vi "manipulate files.vi"(8 "error in":errorcluster) -> (0 "error out":errorcluster)   [LabVIEW 2023]
uses:
  queue/Front Panel Message Queue.lvlib
panel:
  in  "Path to Rename":path
  in  "starting number":i32
  in  "Number to bin":i32
  in  "Path to Bin":path
  in  "binning":bool
  in  "rename":bool
  in  "Stop":bool
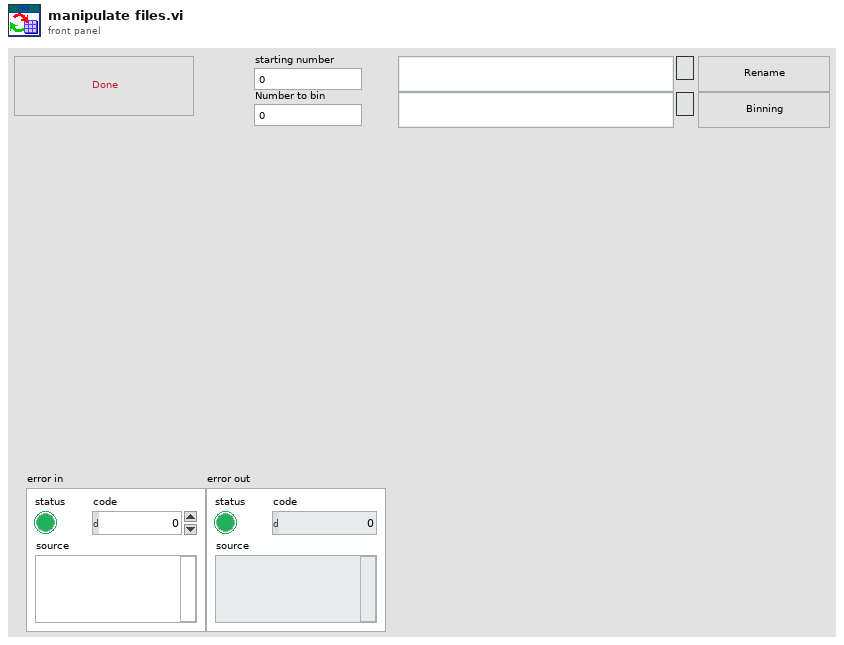
[diagram p1: front panel]
types:
  T1 = typedef "Front Panel Message Queue.lvlib/load Message Queues.ctl" = cluster{"Main":refnum<queue>}
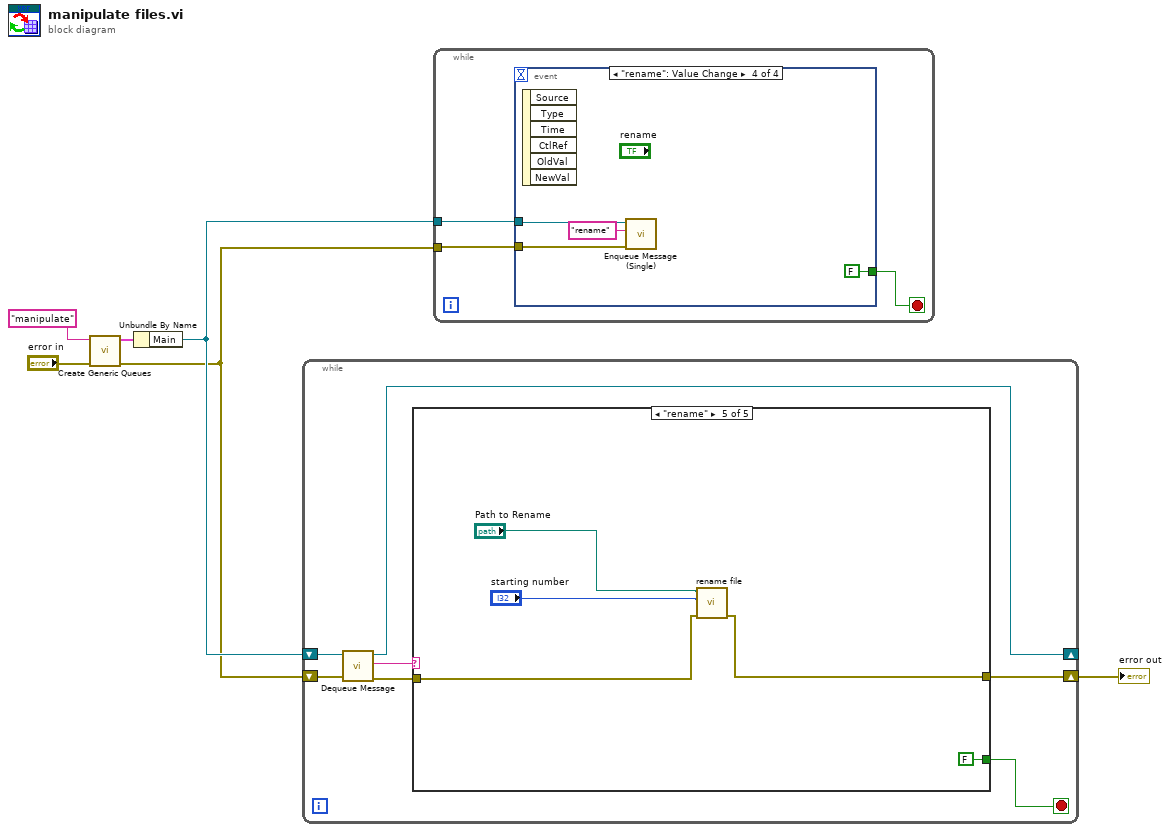
[diagram p0: block diagram]
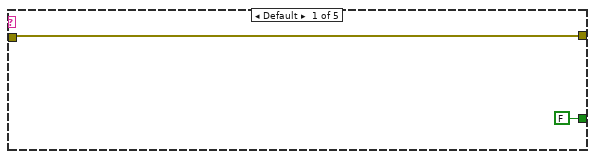
[diagram p2: hidden frame]
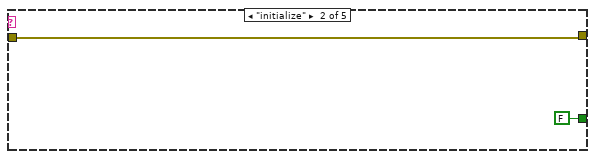
[diagram p3: hidden frame]
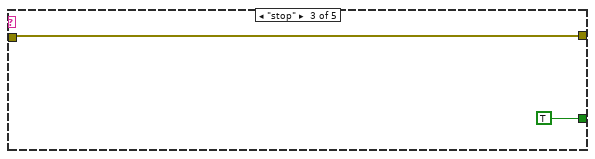
[diagram p4: hidden frame]
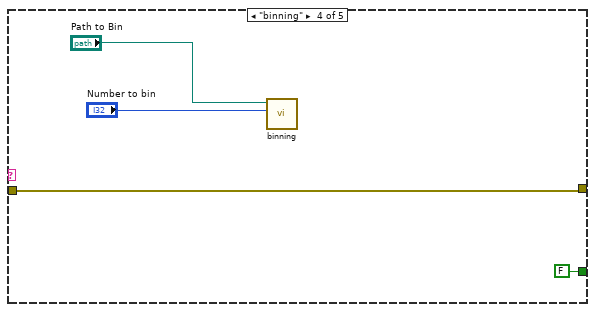
[diagram p5: hidden frame]
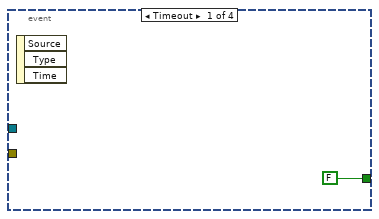
[diagram p6: hidden frame]
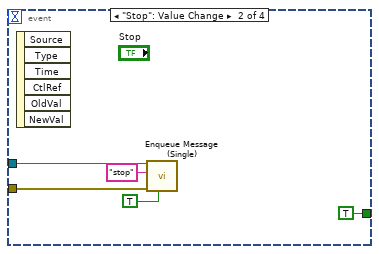
[diagram p7: hidden frame]
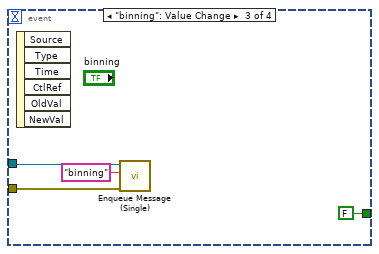
[diagram p8: hidden frame]
diagram:
  n1 = call "Create Generic Queues.vi"("error in (no error)"="error in", "name"="manipulate") -> ("error out"=w2:errorcluster, "Message Queues"=w4:T1)  [unwired: 8 in]
  n2 = Unbundle By Name(w4) -> ("Main"=w3:refnum<queue>)
  n3 = while {
    shift-right: [w10] -> _
    shift-left: w3 -> [w13]
    shift-right: [w9] -> w1
    shift-left: w2 -> [w12]
    stop <- w7 stop-if-true
    n4 = call "Dequeue Message.vi"("error in (no error)"=w12, "Message Queue"=w13) -> ("error out"=w11:errorcluster, "Message"=w8:string, "dup Message Queue"=w10:refnum<queue>)  [unwired: 5 in, 2 out]
    n5 = case shown="\"rename\"" w8 {
      tunnel: w11 -> [w15 w17 w18 w20 w25]
      tunnel: [w15 w17 w18 w20 w24] -> w9
      tunnel: [FALSE FALSE TRUE FALSE FALSE] -> w7
      frame Default {
      }
      frame "initialize" {
      }
      frame "stop" {
      }
      frame "binning" {
        n6 = call "binning.vi"("Number to bin"="Number to bin", "path"="Path to Bin") -> ()  [unwired: 10 in]
      }
      frame "rename" {
        n7 = call "rename file.vi"("error in"=w25, "Starting Number"="starting number", "path"="Path to Rename") -> ("error out"=w24:errorcluster)  [unwired: 8 in]
      }
    }
  }
  "error out" <- w1
  n8 = while {
    tunnel: w3 -> [w30]
    tunnel: w2 -> [w29]
    stop <- w31 stop-if-true
    n9 = event shown="[3] \"rename\": Value Change" {
      selector: _ -> [_ _ _ _]
      dyn-events: _ -> [_ _ _ _]
      timeout: _ -> [_ _ _ _]
      tunnel: [FALSE TRUE FALSE FALSE] -> w31
      tunnel: w30 -> [_ w37 w40 w44]
      tunnel: w29 -> [_ w36 w41 w45]
      event Timeout {
        n10 = event-data() -> ()  [unwired: 1 in, 3 out]
      }
      event "Stop": Value Change {
        n11 = event-data() -> ()  [unwired: 1 in, 6 out]
        n12 = call "Enqueue Message (Single).vi"("Priority Message? (F)"=TRUE, "error in (no error)"=w36, "Message"="stop", "Message Queue"=w37) -> ()  [unwired: 6 in, 2 out]
      }
      event "binning": Value Change {
        n13 = event-data() -> ()  [unwired: 1 in, 6 out]
        n14 = call "Enqueue Message (Single).vi"("error in (no error)"=w41, "Message"="binning", "Message Queue"=w40) -> ()  [unwired: 7 in, 2 out]
      }
      event "rename": Value Change {
        n15 = event-data() -> ()  [unwired: 1 in, 6 out]
        n16 = call "Enqueue Message (Single).vi"("error in (no error)"=w45, "Message"="rename", "Message Queue"=w44) -> ()  [unwired: 7 in, 2 out]
      }
    }
  }
